vi "CRC Logging.vi"(6 "CRC file refnum":refnum<file>, 7 "Input data":u16[](array[numeric]), 8 "CRCH_Rx":u8, 9 "CRCL_Rx":u8, 10 "CRCH":u8, 11 "CRCL":u8) -> (3 "CRC file refnum out":refnum<file>)   [LabVIEW 2020]
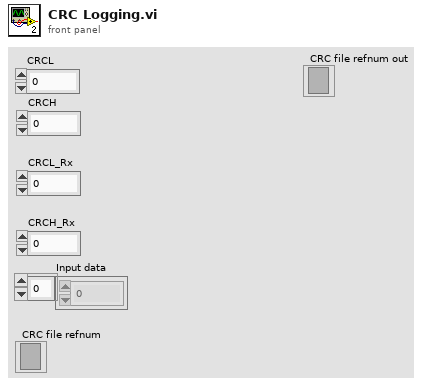
[diagram p1: front panel]
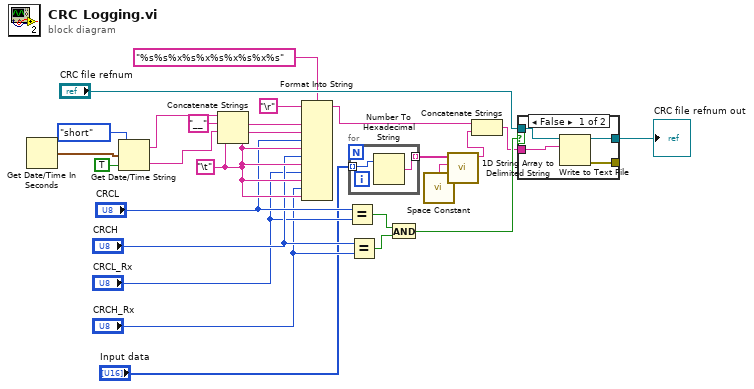
[diagram p0: block diagram]
diagram:
  w22 = "\t"
  n1 = Get Date/Time In Seconds() -> (seconds since 1Jan1904=w19:timestamp)
  n2 = Get Date/Time String(date format (0)=enum16{"short", "long", "abbreviated"}."short", seconds (now)=w19, want seconds? (F)=TRUE) -> (date string=w11:string, time string=w21:string)
  n3 = Concatenate Strings(w11, "__" ("string"), w21, w22) -> (w12:string)
  n4 = Format Into String(format string="%s%s%x%s%x%s%x%s%x%s", initial string="\r", w12, w22, "CRCL", w22, "CRCH", w22, "CRCL_Rx", w22, "CRCH_Rx", w22) -> (resulting string=w17:string)  [unwired: 1 in, 1 out]
  n5 = Equal?(x="CRCL", y="CRCL_Rx") -> (x = y?=w24:bool)
  n6 = for {
    tunnel: "Input data" -> [w27] mode=indexing
    tunnel: [w26] -> w14 mode=indexing
    n7 = Number To Hexadecimal String(2:w27) -> (0:w26:string)  [unwired: 1 in]
  }
  n8 = Equal?(x="CRCH", y="CRCH_Rx") -> (x = y?=w23:bool)
  n9 = And(x=w24, y=w23) -> (x .and. y?=w25:bool)
  n10 = call <vilib>:"Space Constant.vi"() -> ("String"=w15:string)
  n11 = call <vilib>:"1D String Array to Delimited String.vi"("delimiter"=w15, "string array"=w14) -> ("delimited string"=w16:string)  [unwired: 9 in]
  n12 = Concatenate Strings(w17, w16) -> (w18:string)
  n13 = case shown="False" w25 {
    tunnel: w18 -> [w31 _]
    tunnel: "CRC file refnum" -> [w29 w32]
    tunnel: [w30 w32] -> w2
    tunnel: [w28 _] -> _
    frame False {
      n14 = Write to Text File(file (use dialog)=w29, text=w31) -> (refnum out=w30:refnum<file>, error out=w28:errorcluster)  [unwired: 2 in, 1 out]
    }
    frame True {
    }
  }
  "CRC file refnum out" <- w2
